vi "RT main.vi"   [LabVIEW 2017]
uses:
  <vilib>/Platform/TimedLoop/XDataNode/timing_clust.ctl
  <vilib>/Platform/TimedLoop/XDataNode/nitl_modes.ctl
  <vilib>/Platform/TimedLoop/XDataNode/wakeup.ctl
  <vilib>/myRIO/Common/Instrument Driver Framework/myRIO v1.0/UART/vis/myRIO v1.0 Close UART.vi
  <vilib>/myRIO/Common/Instrument Driver Framework/Utilities/vis/FPGA Ref Manager.vi
  <vilib>/myRIO/Common/Instrument Driver Framework/myRIO v1.0/myRIO v1.0 Reset FPGA.vi
  <vilib>/myRIO/Common/Instrument Driver Framework/myRIO v1.0/IRQ/vis/myRIO v1.0 IRQ Info FGV.vi
  <vilib>/myRIO/Common/Instrument Driver Framework/myRIO v1.0/IRQ/vis/myRIO v1.0 Timer IRQ Info FGV.vi
  <vilib>/myRIO/Common/Instrument Driver Framework/myRIO v1.0/IRQ/vis/myRIO v1.0 ISR Agent.vi
  <vilib>/platform/TimedLoop/XDataNode/XDataNode.xnode
  <vilib>/Platform/TimedLoop/XDataNode/XDNodeRunTimeDep.lvlib
  <vilib>/myRIO/Instrument Drivers/Utilities/Utilities.lvlib
types:
  T1 = typedef "XDNodeRunTimeDep.lvlib/timing_clust.ctl" = cluster{"Expected End [f-1]":u64, "Actual End [f-1]":u64, "Finished Late? [f-1]":bool, "Expected End [i-1]":u64, "Actual End [i-1]":u64, "Finished Late? [i-1]":bool, "Expected Start [i]":u64, "Actual Start [i]":u64, "Expected Start [f]":u64, "Actual Start [f]":u64, "Source Name":string, "Structure Name":string, "Period":i64, "Deadline":i64, "Offset":i64, "Start":i64, "Priority":i32, "Timeout":i32, "Mode":T2, "Wakeup Reason":T3, "Error":errorcluster, "Source Type":string, "Secondary Source Type":string, "Global End Time":u64, "Global Start Time":u64, "Frame Duration":u64, "Iteration Duration":u64, "Assigned CPU":i32, "I/O Scan Engine Mode":u32}
  T2 = typedef "XDNodeRunTimeDep.lvlib/nitl_modes.ctl" = enum32{"No Change", "Process missed periods, maintain original phase", "Discard missed periods, maintain original phase", "Process missed periods, ignore original phase", "Discard missed periods, ignore original phase"}
  T3 = typedef "XDNodeRunTimeDep.lvlib/wakeup.ctl" = enum32{"Normal", "Aborted", "Asynchronous wakeup", "Timing source error", "Timed loop error", "Timeout"}
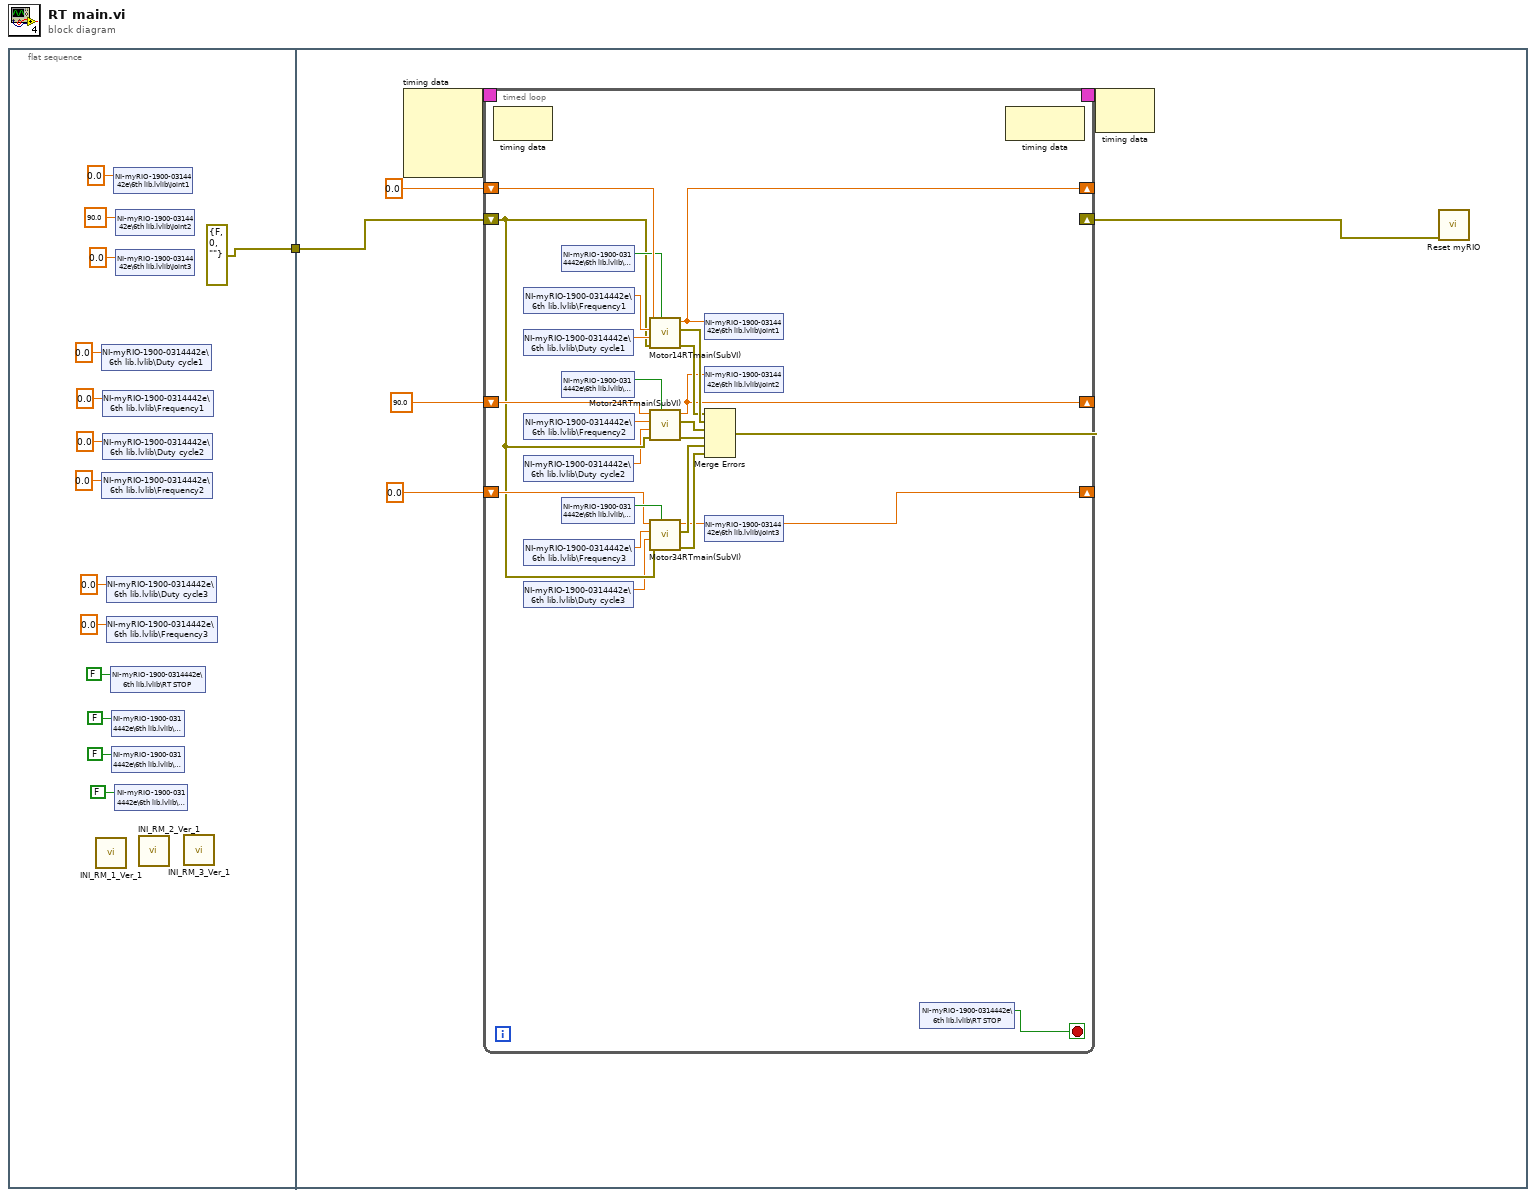
[diagram p0: block diagram]
diagram:
  n1 = flat-sequence {
    tunnel: [errorcluster {"status"=FALSE, "code"=0, "source"=""} ("error in (no error)")] -> w1
    tunnel: w1 -> [w19]
    frame #0 {
      n2 = call "INI_RM_1_Ver_1.vi"() -> ()  [unwired: 12 in]
      n3 = shared-variable "NI-myRIO-1900-0314442e\\6th lib.lvlib\\Duty cycle1"(0.0 ("Duty cycle")) -> ()  [unwired: 1 in, 1 out]
      n4 = shared-variable "NI-myRIO-1900-0314442e\\6th lib.lvlib\\Frequency2"(0.0 ("Frequency2")) -> ()  [unwired: 1 in, 1 out]
      n5 = shared-variable "NI-myRIO-1900-0314442e\\6th lib.lvlib\\Frequency1"(0.0 ("Frequency")) -> ()  [unwired: 1 in, 1 out]
      n6 = shared-variable "NI-myRIO-1900-0314442e\\6th lib.lvlib\\Duty cycle2"(0.0 ("Duty cycle2")) -> ()  [unwired: 1 in, 1 out]
      n7 = shared-variable "NI-myRIO-1900-0314442e\\6th lib.lvlib\\Duty cycle3"(0.0 ("Duty cycle3")) -> ()  [unwired: 1 in, 1 out]
      n8 = shared-variable "NI-myRIO-1900-0314442e\\6th lib.lvlib\\Frequency3"(0.0 ("Frequency3")) -> ()  [unwired: 1 in, 1 out]
      n9 = shared-variable "NI-myRIO-1900-0314442e\\6th lib.lvlib\\RT STOP"(FALSE ("RT STOP")) -> ()  [unwired: 1 in, 1 out]
      n10 = shared-variable "NI-myRIO-1900-0314442e\\6th lib.lvlib\\DIR1"(FALSE ("DIR")) -> ()  [unwired: 1 in, 1 out]
      n11 = shared-variable "NI-myRIO-1900-0314442e\\6th lib.lvlib\\DIR2"(FALSE ("DIR2")) -> ()  [unwired: 1 in, 1 out]
      n12 = shared-variable "NI-myRIO-1900-0314442e\\6th lib.lvlib\\Joint1"(0.0 ("Joint1")) -> ()  [unwired: 1 in, 1 out]
      n13 = shared-variable "NI-myRIO-1900-0314442e\\6th lib.lvlib\\DIR3"(FALSE ("DIR3")) -> ()  [unwired: 1 in, 1 out]
      n14 = shared-variable "NI-myRIO-1900-0314442e\\6th lib.lvlib\\Joint2"(90.0 ("Joint2")) -> ()  [unwired: 1 in, 1 out]
      n15 = shared-variable "NI-myRIO-1900-0314442e\\6th lib.lvlib\\Joint3"(0.0 ("Joint3")) -> ()  [unwired: 1 in, 1 out]
      n16 = call "INI_RM_2_Ver_1.vi"() -> ()  [unwired: 12 in]
      n17 = call "INI_RM_3_Ver_1.vi"() -> ()  [unwired: 12 in]
    }
    frame #1 {
      n18 = node-c288() -> (w22:T1)  [unwired: 4 in]
      n19 = timed-loop {
        timing: w22 -> [_]
        timing-out: [_] -> w21
        shift-right: [w44] -> w20
        shift-left: w19 -> [w31]
        shift-right: [w40] -> _
        shift-left: 0.0 -> [w42]
        shift-right: [w28] -> _
        shift-left: 90.0 -> [w37]
        shift-right: [w27] -> _
        shift-left: 0.0 -> [w32]
        stop <- w43 stop-if-true
        n20 = node-c288() -> ()  [unwired: 1 in, 1 out]
        n21 = shared-variable "NI-myRIO-1900-0314442e\\6th lib.lvlib\\Frequency1"() -> (w41:dbl)  [unwired: 1 in, 1 out]
        n22 = shared-variable "NI-myRIO-1900-0314442e\\6th lib.lvlib\\Duty cycle1"() -> (w38:dbl)  [unwired: 1 in, 1 out]
        n23 = shared-variable "NI-myRIO-1900-0314442e\\6th lib.lvlib\\Frequency2"() -> (w26:dbl)  [unwired: 1 in, 1 out]
        n24 = shared-variable "NI-myRIO-1900-0314442e\\6th lib.lvlib\\Duty cycle2"() -> (w25:dbl)  [unwired: 1 in, 1 out]
        n25 = shared-variable "NI-myRIO-1900-0314442e\\6th lib.lvlib\\Frequency3"() -> (w24:dbl)  [unwired: 1 in, 1 out]
        n26 = shared-variable "NI-myRIO-1900-0314442e\\6th lib.lvlib\\Duty cycle3"() -> (w23:dbl)  [unwired: 1 in, 1 out]
        n27 = shared-variable "NI-myRIO-1900-0314442e\\6th lib.lvlib\\DIR1"() -> (w39:bool)  [unwired: 1 in, 1 out]
        n28 = shared-variable "NI-myRIO-1900-0314442e\\6th lib.lvlib\\DIR2"() -> (w36:bool)  [unwired: 1 in, 1 out]
        n29 = shared-variable "NI-myRIO-1900-0314442e\\6th lib.lvlib\\DIR3"() -> (w33:bool)  [unwired: 1 in, 1 out]
        n30 = call "Motor14RTmain(SubVI).vi"("Boolean"=w39, "error in (no error)"=w31, "Double"=w38, "Double 2"=w41, "Numeric in"=w42) -> ("error out"=w45:errorcluster, "error out 2"=w46:errorcluster, "Numeric out"=w40:dbl)  [unwired: 4 in]
        n31 = call "Motor24RTmain(SubVI).vi"("Boolean"=w36, "error in (no error)"=w31, "Double"=w25, "Double 2"=w26, "Numeric in"=w37) -> ("error out"=w34:errorcluster, "error out 2"=w35:errorcluster, "Numeric out"=w28:dbl)  [unwired: 4 in]
        n32 = call "Motor34RTmain(SubVI).vi"("Boolean"=w33, "error in (no error)"=w31, "Double"=w23, "Double 2"=w24, "Numeric in"=w32) -> ("error out"=w29:errorcluster, "error out 2"=w30:errorcluster, "Numeric out"=w27:dbl)  [unwired: 4 in]
        n33 = shared-variable "NI-myRIO-1900-0314442e\\6th lib.lvlib\\Joint1"(w40) -> ()  [unwired: 1 in, 1 out]
        n34 = shared-variable "NI-myRIO-1900-0314442e\\6th lib.lvlib\\Joint2"(w28) -> ()  [unwired: 1 in, 1 out]
        n35 = Merge Errors(w45, w46, w35, w34, w30, w29) -> (w44:errorcluster)
        n36 = shared-variable "NI-myRIO-1900-0314442e\\6th lib.lvlib\\Joint3"(w27) -> ()  [unwired: 1 in, 1 out]
        n37 = shared-variable "NI-myRIO-1900-0314442e\\6th lib.lvlib\\RT STOP"() -> (w43:bool)  [unwired: 1 in, 1 out]
        n38 = node-c288() -> ()  [unwired: 1 in, 1 out]
      }
      n39 = node-c288(w21) -> ()  [unwired: 1 out]
      n40 = call <vilib>:"Reset myRIO.vi"("error in (no error)"=w20) -> ()  [unwired: 10 in, 1 out]
    }
  }
